vi "FINAL.vi"() -> ()   [LabVIEW 2015]
uses:
  <vilib>/httpClient/LabVIEWHTTPClient.lvlib
  <vilib>/MakerHub/LINX/LMH-LINX.lvlib
panel:
  in  "String":string="http://apidev.accuweather.com/forecasts/v1/hourly/12hour/6788_PC?apikey=c3e7df4f2d6a40698cc75fac1b6a2c83&language=en&details=false&metric=false"
  in  "Run Again":bool
  in  "stop":bool
  in  "Port List":i32[](array[numeric])
  in  "Serial Port":refnum<visa-resource-name>="N/A"
  out "Arduino Input":bool[](array[boolean])
  in  "BOOL Array Input":bool[](array[boolean])
  out "IsRain?":bool
  out "IsCold":dbl
  out "Temperature Average":dbl
  out "Icon Phrases":string[](array[string])
  out "Icon Phrase Indexes":i32[](array[numeric])
  out "Temperature Values Output":i32[](array[numeric])
  out "Values Indexes":i32[](array[numeric])
  out "Temperature Indexes":i32[](array[numeric])
  out "Array":string[](array[string])
  out "Variable Names":string[](array[string])
  out "Token Array":T1(array[ring])
  out "body":string
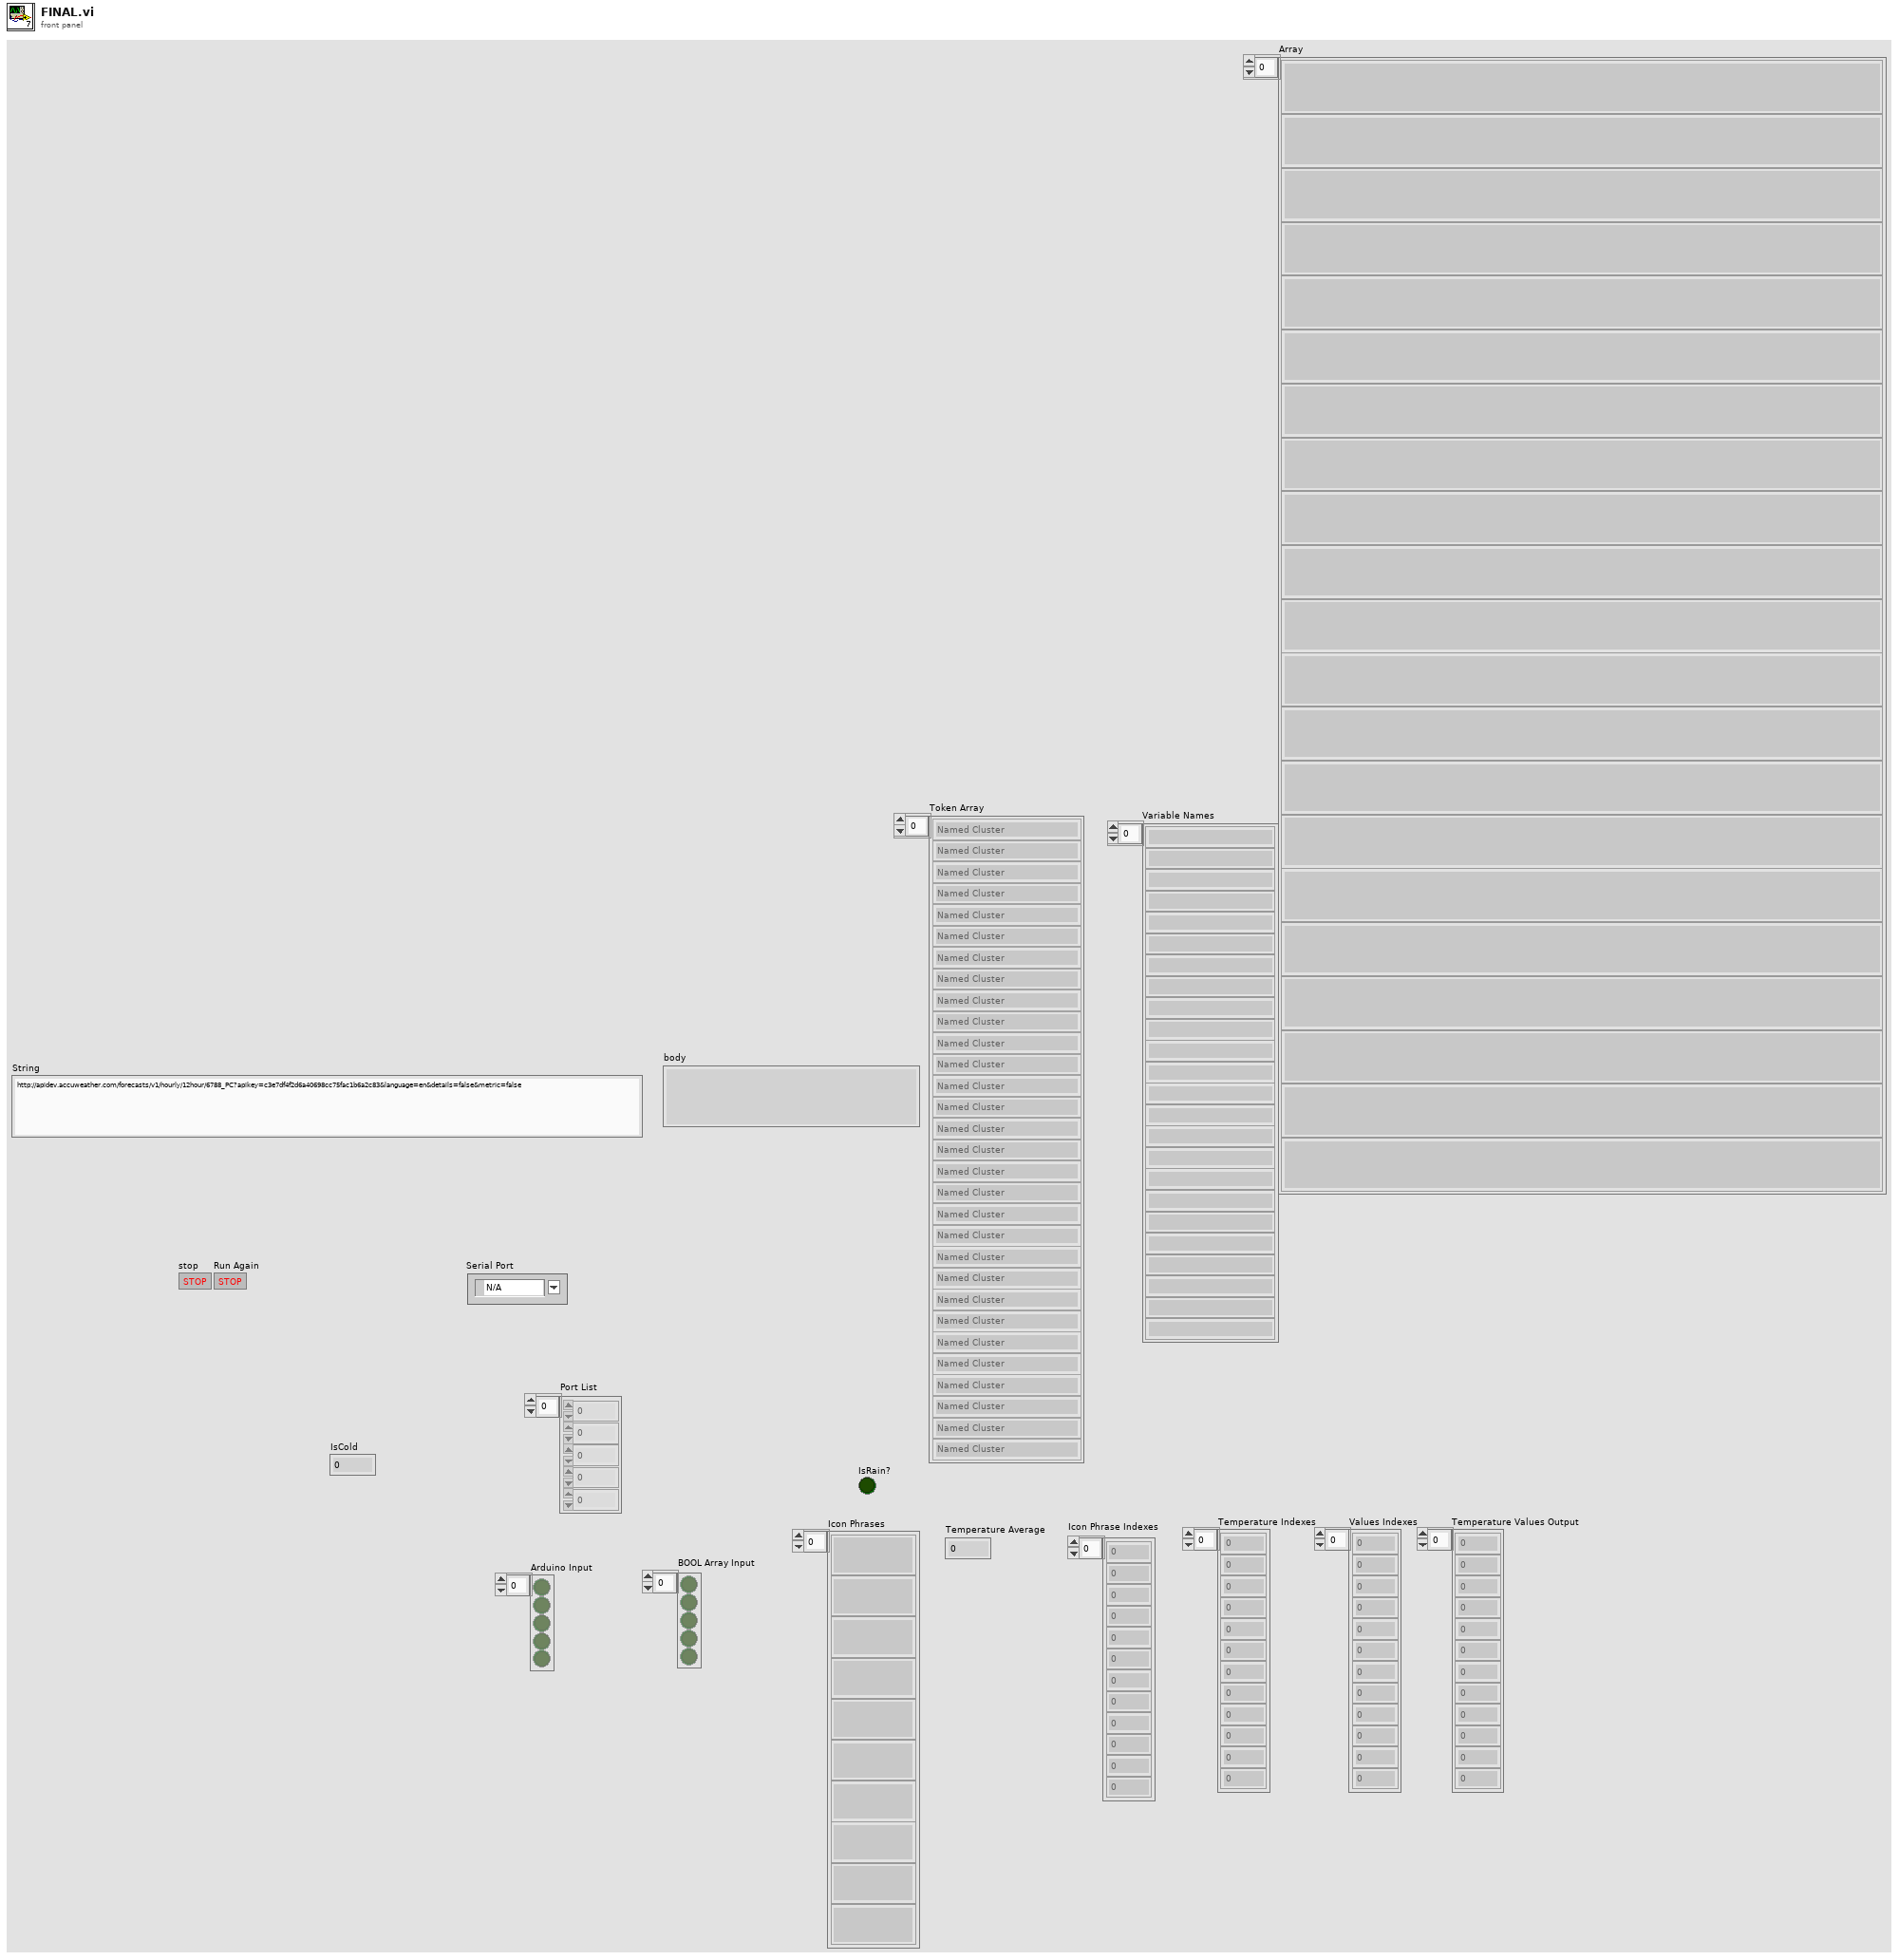
[diagram p1: front panel]
types:
  T1 = enum16{"End", "Boolean", "Named Cluster", "Unnamed Cluster", "Array", "String", "Decimal", "FloatingPoint", "End Array", "End Cluster"}[]
  T2 = typedef "LMH-LINX.lvlib/LINX Ref.ctl" = cluster{"Platform":T3, "Interface":T4, "LINX Device Config":T5}
  T3 = typedef "LMH-LINX.lvlib/Platform.ctl" = enum16{"LINX", "myRIO"}
  T4 = typedef "LMH-LINX.lvlib/Interface.ctl" = enum16{"Serial", "TCP"}
  T5 = typedef "LMH-LINX.lvlib/Device.lvlib/LINX Device Config.ctl" = cluster{"Interface":T4, "COM Port":refnum<visa-resource-name>, "TCP Configuration":T6, "Device Family":u8, "Device ID":u8, "Device Name":string, "TCP Ref":refnum<k5>, "Channels":T7}
  T6 = typedef "LMH-LINX.lvlib/Device.lvlib/TCP Config.ctl" = cluster{"IP Address":string, "Port":u16}
  T7 = typedef "LMH-LINX.lvlib/Channels.ctl" = cluster{"DI":u8[], "DO":u8[], "AI":u8[], "AO":u8[], "PWM":u8[], "QE":u8[], "UART":u8[], "I2C 2":u8[], "SPI":u8[], "CAN":u8[], "Servo":u8[], "AI Ref (V)":dbl, "AO Ref (V)":dbl, "AO Resolution (Bits)":u8}
  T8 = typedef "LabVIEWHTTPClient.lvlib/ClientHandle.ctl" = refnum<k1>
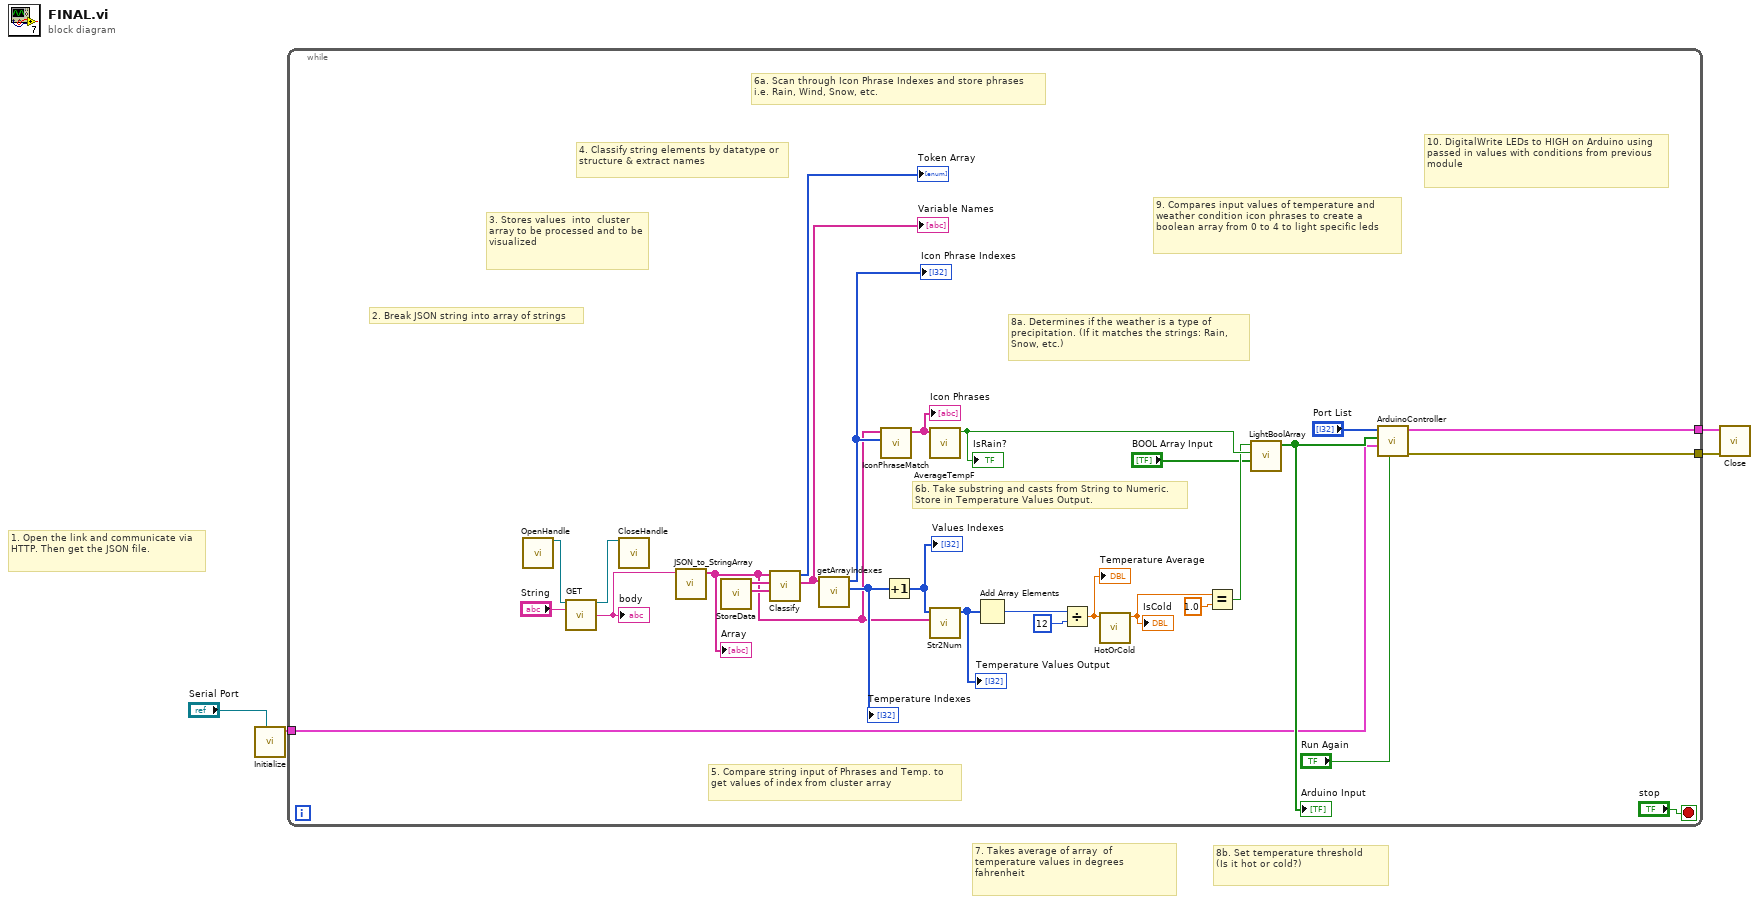
[diagram p0: block diagram]
diagram:
  # "8b. Set temperature threshold \n(Is it hot or cold?)"
  # "7. Takes average of array  of temperature values in degrees fahrenheit"
  # "1. Open the link and communicate via HTTP. Then get the JSON file."
  n1 = call <vilib>:"Initialize.vi"("Serial Port"="Serial Port") -> ("LINX Ref"=w3:T2)  [unwired: 8 in, 2 out]
  n2 = while {
    tunnel: w3 -> [w10]
    tunnel: [w9] -> w2
    tunnel: [w8] -> w1
    stop <- "stop" stop-if-true
    # "5. Compare string input of Phrases and Temp. to get values of index from cluster array"
    # "2. Break JSON string into array of strings"
    # "3. Stores values  into  cluster array to be processed and to be visualized"
    # "4. Classify string elements by datatype or structure & extract names"
    # "9. Compares input values of temperature and weather condition icon phrases to create a boolean array from 0 to 4 to light specific leds"
    # "6a. Scan through Icon Phrase Indexes and store phrases\ni.e. Rain, Wind, Snow, etc."
    # "8a. Determines if the weather is a type of precipitation. (If it matches the strings: Rain, Snow, etc.)"
    # "10. DigitalWrite LEDs to HIGH on Arduino using passed in values with conditions from previous module"
    # "6b. Take substring and casts from String to Numeric. \nStore in Temperature Values Output."
    n3 = call <vilib>:"OpenHandle.vi"() -> ("client handle out"=w33:T8)  [unwired: 14 in, 1 out]
    n4 = call <vilib>:"GET.vi"("client handle"=w33, "url"="String") -> ("client handle out"=w32:T8, "body"=w28:string)  [unwired: 10 in, 2 out]
    "body" <- w28
    n5 = call <vilib>:"CloseHandle.vi"("client handle"=w32) -> ()  [unwired: 14 in, 1 out]
    n6 = call "JSON_to_StringArray.vi"("body"=w28) -> ("Array"=w13:string[])  [unwired: 10 in]
    "Array" <- w13
    n7 = call "StoreData.vi"() -> ("Array"=w29:string[], "delimiters"=w31:string[])  [unwired: 10 in]
    n8 = call "Classify.vi"("Array 3"=w29, "delimiters"=w31, "Array in"=w13) -> ("Array out"=w14:string[], "Array 4"=→"Token Array":T1)  [unwired: 7 in]
    "Variable Names" <- w14
    n9 = call "getArrayIndexes.vi"("Array in"=w14) -> ("Array 2"=w27:i32[], "Array"=w26:i32[])  [unwired: 9 in]
    "Temperature Indexes" <- w27
    "Icon Phrase Indexes" <- w26
    n10 = call "IconPhraseMatch.vi"("Array 3"=w26, "Array in"=w13) -> ("Array out"=w22:string[])  [unwired: 9 in]
    "Icon Phrases" <- w22
    n11 = Increment(x=w27) -> (x+1=w5:i32[])
    "Values Indexes" <- w5
    n12 = call "AverageTempF.vi"("Array"=w22) -> ("Boolean"=w18:bool)  [unwired: 10 in]
    "IsRain?" <- w18
    n13 = call "Str2Num.vi"("Array in"=w13, "Array 3"=w5) -> ("Array out"=w25:i32[])  [unwired: 9 in]
    "Temperature Values Output" <- w25
    n14 = Add Array Elements(numeric array=w25) -> (sum=w24:i32)
    n15 = Divide(x=w24, y=12) -> (x/y=w21:dbl)
    "Temperature Average" <- w21
    n16 = call "HotOrCold.vi"("Numeric"=w21) -> ("cold"=w20:dbl)  [unwired: 10 in]
    "IsCold" <- w20
    n17 = Equal?(x=w20, y=1.0) -> (x = y?=w17:bool)
    n18 = call "LightBoolArray.vi"("BOOL Array Input in"="BOOL Array Input", "Boolean 2"=w18, "Boolean"=w17) -> ("BOOL Array Input out"=w12:bool[])  [unwired: 8 in]
    "Arduino Input" <- w12
    n19 = call "ArduinoController.vi"("Run Again"="Run Again", "LINX Ref"=w10, "BOOL Array Input"=w12, "Port List"="Port List") -> ("error out"=w8:errorcluster, "LINX Resource"=w9:T2)  [unwired: 6 in]
  }
  n20 = call <vilib>:"Close.vi"("Error In"=w1, "LINX Resource"=w2) -> ()  [unwired: 8 in, 2 out]
